vi "HEWH CloseEquipmet.vi"(7 "Semiphore":T1, 8 "Error In":errorcluster, 11 "Equipment":T2={"COM Port"="COM1", "MW100"="MW100", "AG34970"="A-34972A", "Chamber"="WT500"}) -> (0 "Error Out":errorcluster)   [LabVIEW 2012]
uses:
  EquipReferences.ctl
  Drivers/Agilent 34970/Agilent 34970.lvlib
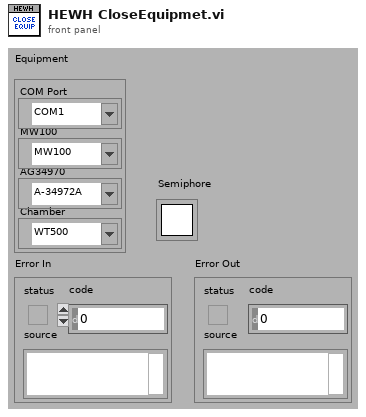
[diagram p1: front panel]
types:
  T1 = typedef "Semaphore RefNum" = refnum<k1>
  T2 = typedef "EquipReferences.ctl" = cluster{"COM Port":refnum<visa-resource-name>, "MW100":refnum<visa-resource-name>, "AG34970":refnum<visa-resource-name>, "Chamber":refnum<visa-resource-name>}
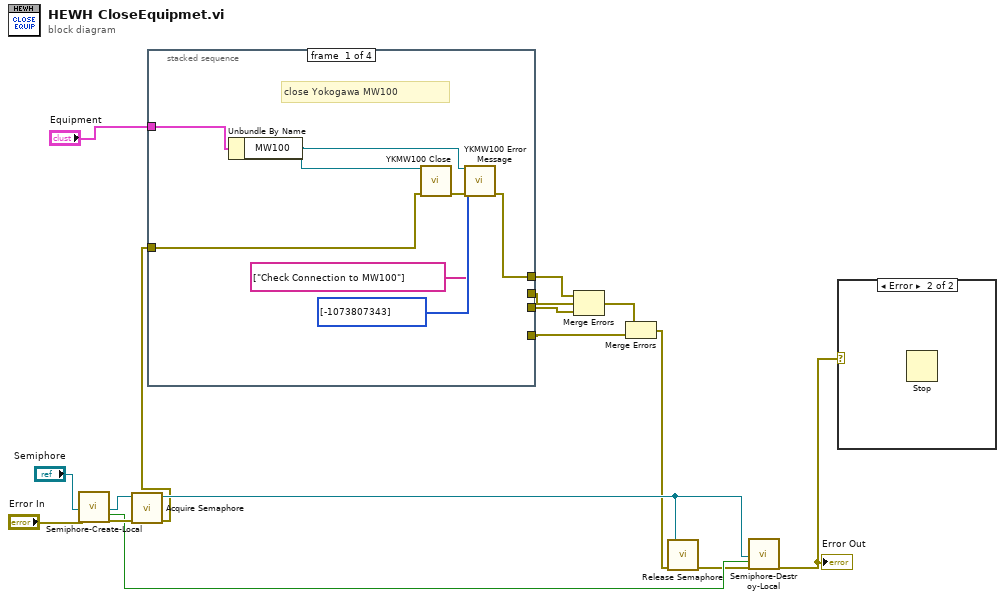
[diagram p0: block diagram]
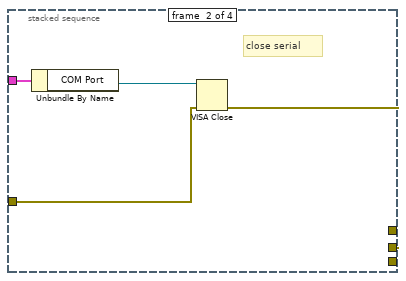
[diagram p3: hidden frame]
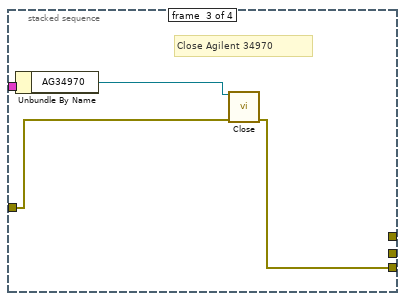
[diagram p4: hidden frame]
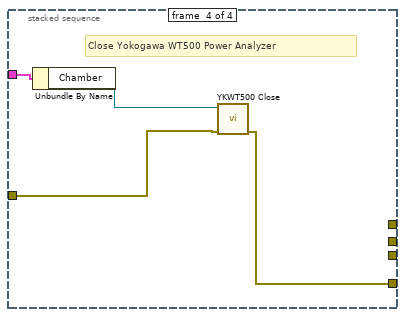
[diagram p5: hidden frame]
diagram:
  n1 = call "Semiphore-Create-Local.vi"("Semiphore"="Semiphore", "error in (no error)"="Error In") -> ("semaphore"=w9:T1, "Local?"=w6:bool, "error out"=w8:errorcluster)  [unwired: 15 in]
  n2 = call <vilib>:"Acquire Semaphore.vi"("error in (no error)"=w8, "semaphore"=w9) -> ("error out"=w3:errorcluster, "semaphore out"=w7:T1)  [unwired: 3 in, 1 out]
  n3 = stacked-sequence {
    tunnel: "Equipment" -> [w23 w27 w31 w35]
    tunnel: [_ _ _ w34] -> w12
    tunnel: w3 -> [w22 w25 w29 w32]
    tunnel: [w20 _ _ _] -> w16
    tunnel: [_ w24 _ _] -> w15
    tunnel: [_ _ w28 _] -> w14
    frame #0 {
      # "close Yokogawa MW100"
      n4 = Unbundle By Name(w23) -> ("MW100"=w19:refnum<visa-resource-name>)
      n5 = call "YKMW100 Close.vi"("VISA session"=w19, "error in (no error)"=w22) -> ("error out"=w21:errorcluster)  [unwired: 13 in]
      n6 = call "YKMW100 Error Message.vi"("VISA session"=w19, "User-Defined Descriptions"=string[] ["Check Connection to MW100"], "User-Defined Codes"=i32[] [-1073807343], "error in (no error)"=w21) -> ("error out"=w20:errorcluster)  [unwired: 7 in, 4 out]
    }
    frame #1 {
      # "close serial"
      n7 = Unbundle By Name(w27) -> ("COM Port"=w26:refnum<visa-resource-name>)
      n8 = VISA Close(VISA resource name=w26, error in (no error)=w25) -> (error out=w24:errorcluster)
    }
    frame #2 {
      # "Close Agilent 34970"
      n9 = Unbundle By Name(w31) -> ("AG34970"=w30:refnum<visa-resource-name>)
      n10 = call "Close.vi"("VISA Resource Name"=w30, "error in (no error)"=w29) -> ("error out"=w28:errorcluster)  [unwired: 13 in]
    }
    frame #3 {
      # "Close Yokogawa WT500 Power Analyzer"
      n11 = Unbundle By Name(w35) -> ("Chamber"=w33:refnum<visa-resource-name>)
      n12 = call "YKWT500 Close.vi"("error in (no error)"=w32, "VISA resource name"=w33) -> ("error out"=w34:errorcluster)  [unwired: 9 in]
    }
  }
  n13 = Merge Errors(w16, w15, w14) -> (w13:errorcluster)
  n14 = Merge Errors(w13, w12) -> (w2:errorcluster)
  n15 = call <vilib>:"Release Semaphore.vi"("error in (no error)"=w2, "semaphore"=w7) -> ("error out"=w5:errorcluster)  [unwired: 4 in, 1 out]
  n16 = call "Semiphore-Destroy-Local.vi"("Semiphore"=w7, "Local?"=w6, "error in (no error)"=w5) -> ("error out"=w1:errorcluster)  [unwired: 16 in]
  "Error Out" <- w1
  n17 = case shown="Error" w1 {
    frame No Error {
    }
    frame Error {
      n18 = Stop() -> ()  [unwired: 1 in]
    }
  }
